vi "ServerConfig.vi"(8 "error in (no error)":errorcluster, 10 "ServerConfig":refnum<class "ServerConfig.lvclass">, 11 "TcpServer in":refnum<class "TcpServer.lvclass">) -> (0 "error out":errorcluster, 3 "TcpServer out":refnum<class "TcpServer.lvclass">)   [LabVIEW 2022 SP3, in "TcpServer.lvlib" / "TcpServer.lvclass"]
uses:
  TcpServer.lvclass
  C:/Users/jakub/repos/gh/sw4sys/lv-tcp-server-sample/LoggingActor/Source/LoggingActor/LoggingActor/LoggingActor.lvclass
  ServerConfig/ServerConfig.lvclass
  ServerConfig/ServerConfig.lvclass/ServerConfig.ctl
  TcpServer.lvclass/TcpServer.ctl
  TcpSocket/Source/TcpSocket/TcpSocket/TcpSocket.lvclass/TcpSocket.ctl
  TcpSocket/Source/TcpSocket/TcpServer/TcpServer.lvclass/TcpServer.ctl
  LoggingActor/Source/LoggingActor/LoggingActor/LoggingActor.lvclass/LoggingActor.ctl
  TcpSocket/Source/TcpSocket/TcpSocket/Write Address.vi
  TcpSocket/Source/TcpSocket/TcpSocket/Write OpenTimeout.vi
  TcpSocket/Source/TcpSocket/TcpSocket/Write Port.vi
  TcpSocket/Source/TcpSocket/TcpSocket/Write ReadMode.vi
  TcpSocket/Source/TcpSocket/TcpSocket/Write ReadTimeout.vi
  TcpSocket/Source/TcpSocket/TcpSocket/Write WriteTimeout.vi
  TcpSocket/Source/TcpSocket/TcpServer/Write ConnectionTimeout.vi
  ServerConfig/Read Address.vi
  ServerConfig/Read OpenTimeout.vi
  ServerConfig/Read Port.vi
  ServerConfig/Read ReadMode.vi
  ServerConfig/Read ReadTimeout.vi
  ServerConfig/Read WriteTimeout.vi
  ServerConfig/Read ConnectionTimeout.vi
  LoggingActor/Source/LoggingActor/LoggingActor/Read Logger.vi
  TcpSocket/Source/TcpSocket/TcpServer/TcpServer.lvclass
  C:/Users/jakub/repos/gh/sw4sys/lv-tcp-server-sample/TcpSocket/Source/TcpSocket/TcpSocket/TcpSocket.lvclass
  Logger/Source/Logger/Logger.lvclass
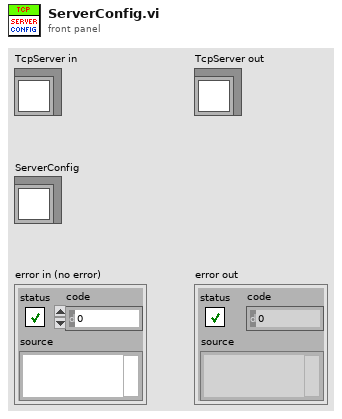
[diagram p1: front panel]
types:
  T1 = enum16{"Standard", "Buffered", "CRLF", "Immediate"}
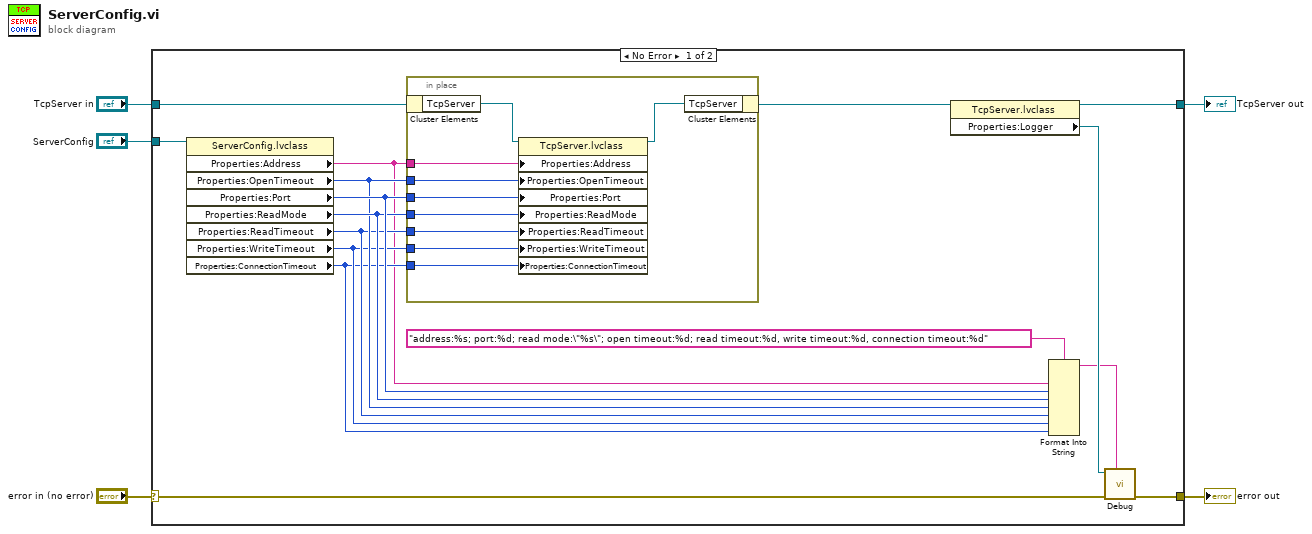
[diagram p0: block diagram]
diagram:
  n1 = case shown="No Error" "error in (no error)" {
    selector: "error in (no error)" -> [w21 w32]
    tunnel: [w18 w32] -> w4
    tunnel: [w17 w31] -> w2
    tunnel: "TcpServer in" -> [w20 w31]
    tunnel: "ServerConfig" -> [w15 _]
    frame No Error {
      n2 = property class="ServerConfig.lvclass"(reference=w15) -> ("Properties:Address"=w8:string, "Properties:OpenTimeout"=w12:i32, "Properties:Port"=w14:u16, "Properties:ReadMode"=w13:T1, "Properties:ReadTimeout"=w11:i32, "Properties:WriteTimeout"=w10:i32, "Properties:ConnectionTimeout"=w9:i32)  [unwired: 1 in, 2 out]
      n3 = in-place {
        in-place-border: w8 -> [w28]
        in-place-border: w12 -> [w27]
        in-place-border: w14 -> [w26]
        in-place-border: w13 -> [w25]
        in-place-border: w11 -> [w24]
        in-place-border: w10 -> [w23]
        in-place-border: w9 -> [w22]
        n4 = in-place-cluster #1(w20) -> ("TcpServer"=w30:refnum<class "TcpServer.lvclass">)
        n5 = property class="TcpServer.lvclass"(reference=w30, "Properties:Address"=w28, "Properties:OpenTimeout"=w27, "Properties:Port"=w26, "Properties:ReadMode"=w25, "Properties:ReadTimeout"=w24, "Properties:WriteTimeout"=w23, "Properties:ConnectionTimeout"=w22) -> (reference out=w29:refnum<class "TcpServer.lvclass">)  [unwired: 1 in, 1 out]
        n6 = in-place-cluster #1("TcpServer"=w29) -> (w19:refnum<class "TcpServer.lvclass">)
      }
      n7 = property class="TcpServer.lvclass"(reference=w19) -> (reference out=w17:refnum<class "TcpServer.lvclass">, "Properties:Logger"=w16:refnum<class "Logger.lvclass">)  [unwired: 1 in, 1 out]
      n8 = Format Into String(format string="address:%s; port:%d; read mode:\"%s\"; open timeout:%d; read timeout:%d, write timeout:%d, connection timeout:%d", w8, w14, w13, w12, w11, w10, w9) -> (resulting string=w7:string)  [unwired: 2 in, 1 out]
      n9 = call-dynamic "Debug.vi"("Message"=w7, "error in (no error)"=w21, "Logger in"=w16) -> ("error out"=w18:errorcluster)  [unwired: 5 in, 1 out]
    }
    frame Error {
    }
  }
  "error out" <- w4
  "TcpServer out" <- w2
